vi "multicolor creation fast-3 only2ch(subvi).vi"(4 "on/off":bool[](array[boolean])=[TRUE, TRUE, FALSE, FALSE, FALSE, FALSE], 5 "colors":T1(array[cluster])=[{"color array"=[0, 16448250, 16448250, 16448250, 16776960, 16711680, 16448250, 16448250], "num of colors"=2, "max"=600.0, "min"=0.0}, {"color array"=[0, 16711680, 16776960, 16448250, 16776960, 16711680, 16448250, 16448250], "num of colors"=2, "max"=2000.0100000000002, "min"=100.0}, {"color array"=[0, 16711680, 16448250, 16448250, 16776960, 16711680, 16448250, 16448250], "num of colors"=2, "max"=12500.0, "min"=0.0}, {"color array"=[0, 255, 16448250, 16448250, 16776960, 16711680, 16448250, 16448250], "num of colors"=2, "max"=1.01, "min"=0.0}, {"color array"=[0, 65280, 16448250, 16448250, 16776960, 16711680, 16448250, 16448250], "num of colors"=3, "max"=1.0, "min"=0.0}, {"color array"=[0, 255, 16448250, 16448250, 16776960, 16711680, 16448250, 16448250], "num of colors"=2, "max"=1.0099999999999991, "min"=0.0}] {"min" step=0.01 format="%_2f"; "max" step=0.1 format="%_3f"}, 8 "fast/slow":bool=TRUE, 9 "img array in":dbl[][][](array[numeric])=array2x1024x1280[2621440 elements]) -> (1 "mixed img array":u32[][](array[numeric]))   [LabVIEW 2024]
panel:
  out "x-y 2":dbl
  out "Array":u32[][](array[numeric])
  out "x-y":dbl
  out "variant":variant
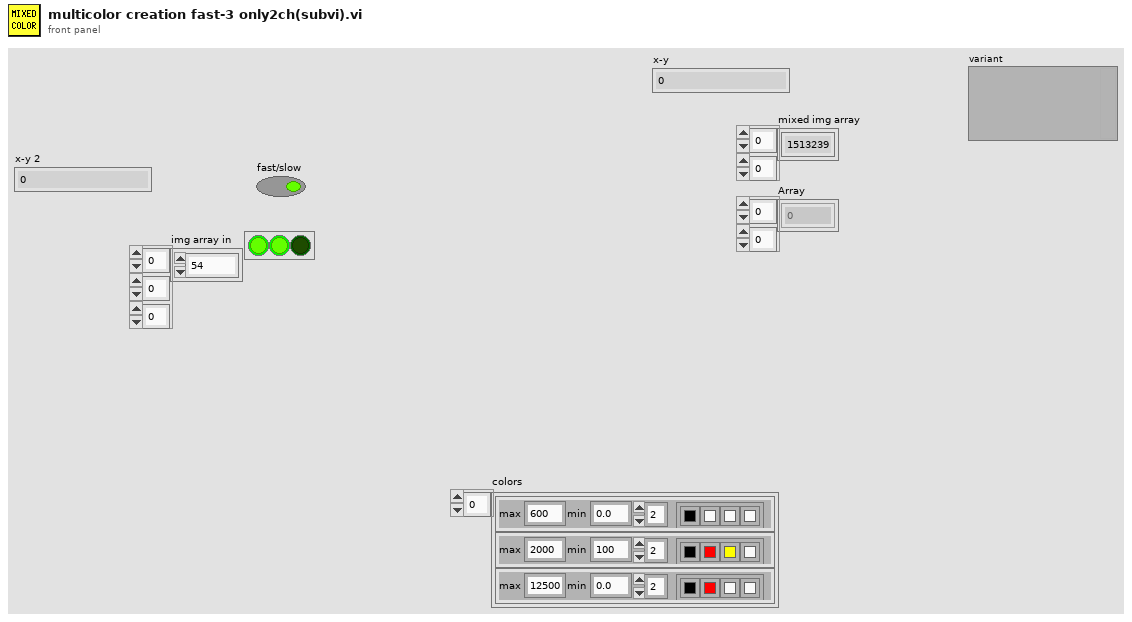
[diagram p1: front panel]
types:
  T1 = cluster{"color array":u32[], "num of colors":i32, "max":dbl, "min":dbl}[]
  T2 = cluster{"color array":u32[], "num of colors":i32, "max":dbl, "min":dbl}
  T3 = cluster{"color array":u32[], "num of colors":i32, "color array":u32[], "num of colors":i32}
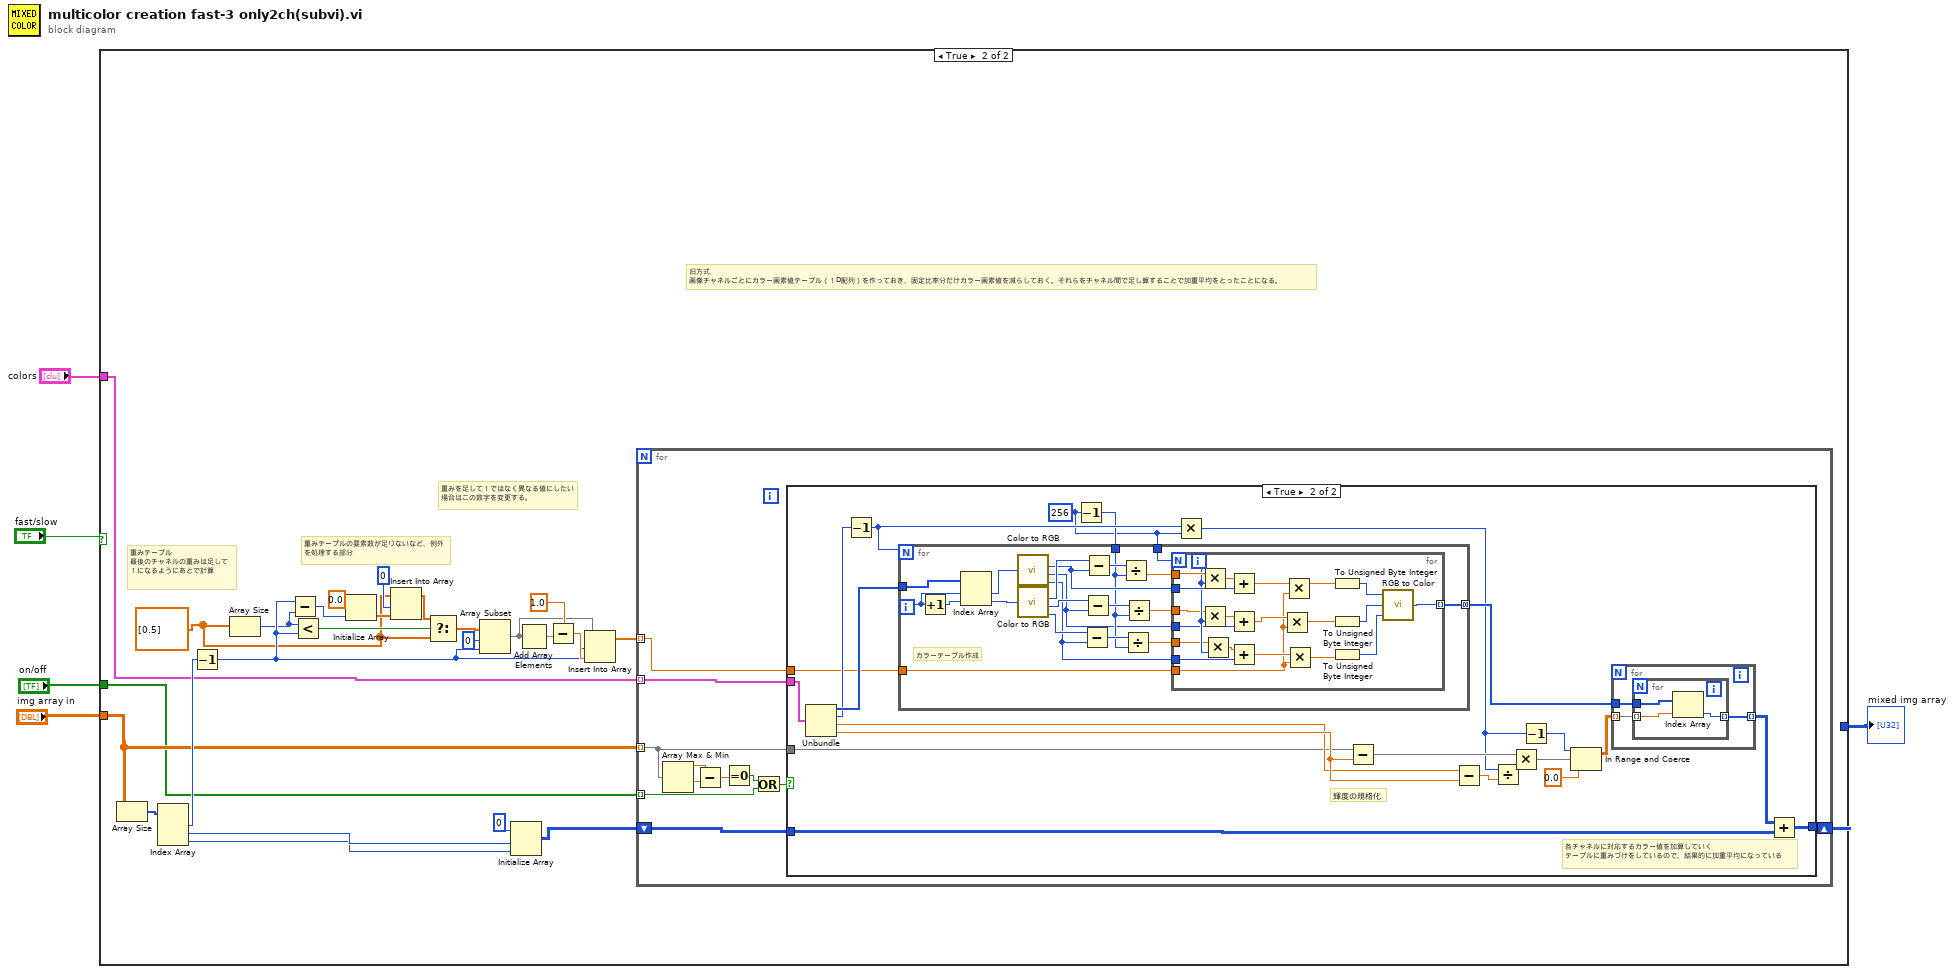
[diagram p0: block diagram]
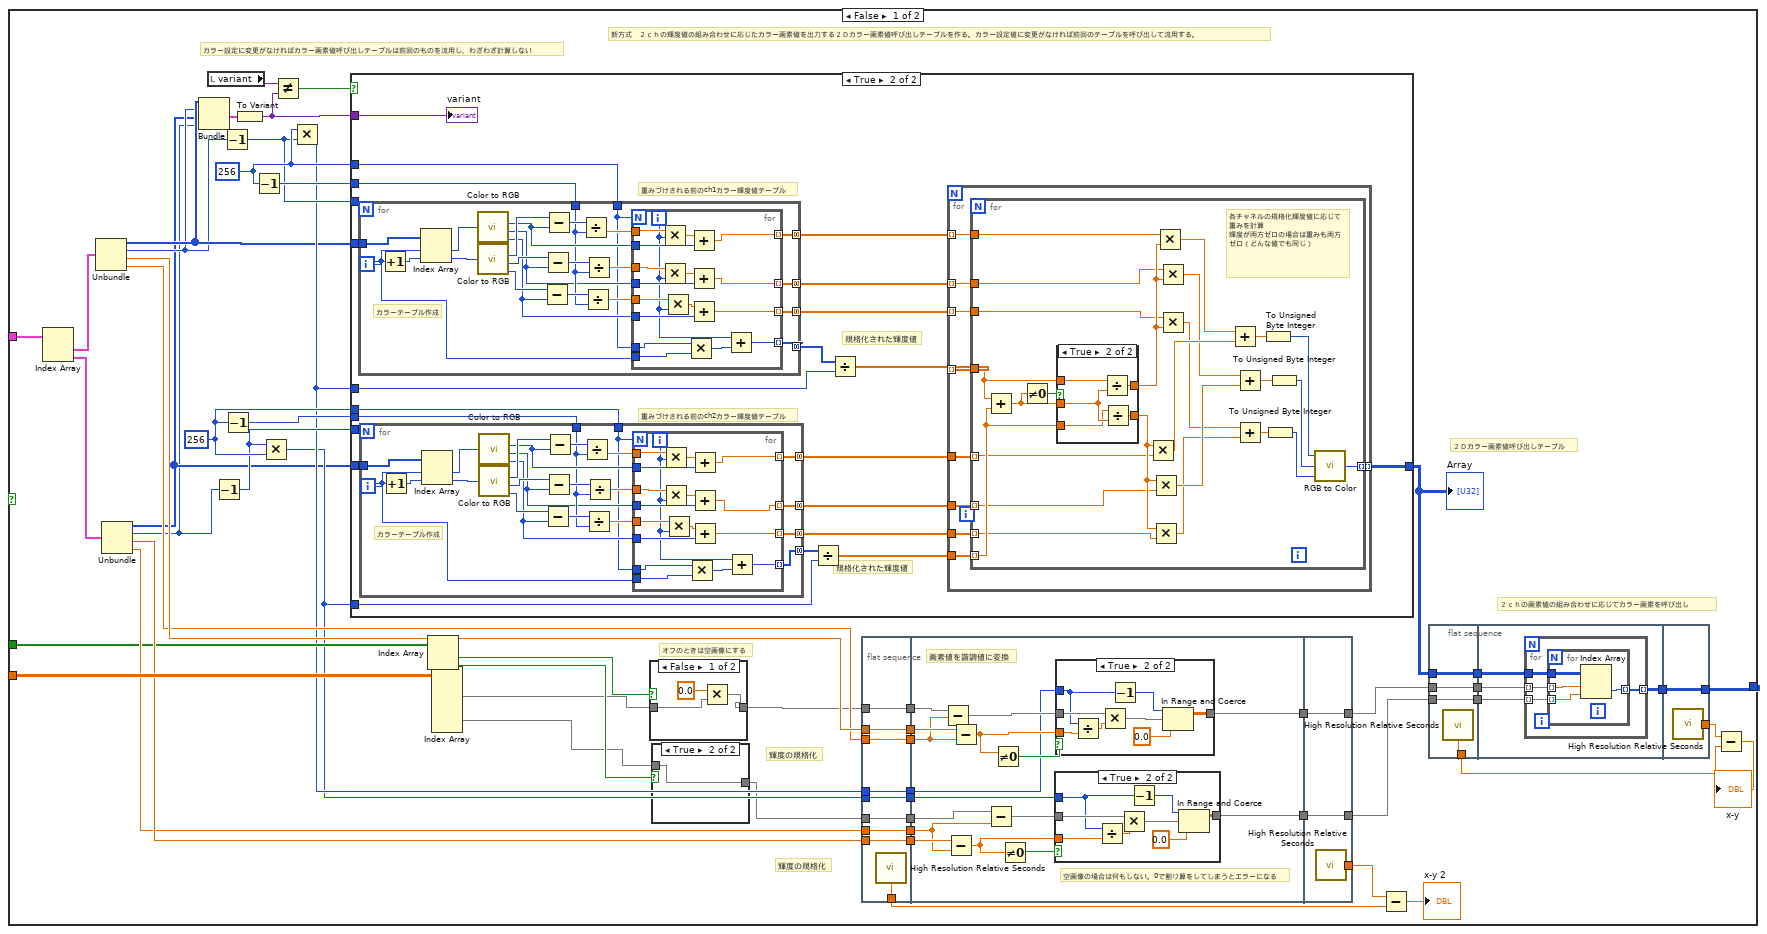
[diagram p2: hidden frame]
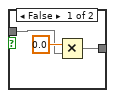
[diagram p3: hidden frame]
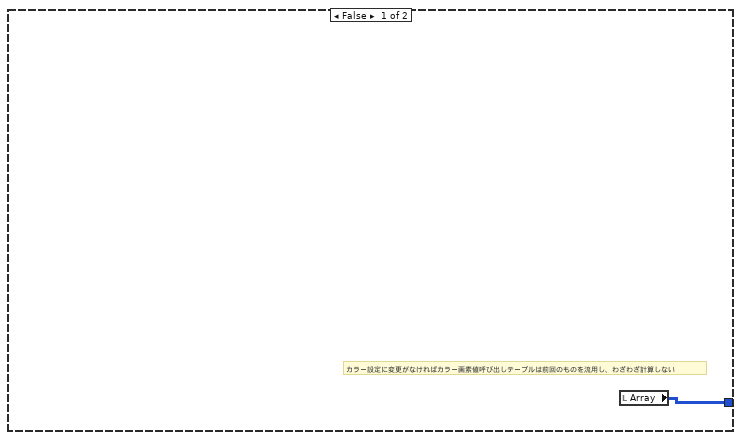
[diagram p7: hidden frame]
diagram:
  n1 = case shown="True" "fast/slow" {
    tunnel: "colors" -> [w46 w280]
    tunnel: "img array in" -> [w41 w279]
    tunnel: [w30 w281] -> w3
    tunnel: "on/off" -> [w29 w278]
    frame False {
      w36 = u16 256 ("y")
      w38 = u16 256 ("y")
      # "カラー設定に変更がなければカラー画素値呼び出しテーブルは前回のものを流用し、わざわざ計算しない"
      # "２ｃｈの画素値の組み合わせに応じてカラー画素を呼び出し"
      # "オフのときは空画像にする"
      # "２Ｄカラー画素値呼び出しテーブル"
      # "新方式　２ｃｈの輝度値の組み合わせに応じたカラー画素値を出力する２Ｄカラー画素値呼び出しテーブルを作る。カラー設定値に変更がなければ前回のテーブルを呼び出して流用する。"
      # "輝度の規格化"
      # "輝度の規格化"
      n2 = Index Array(array=w46) -> (element #1=w44:T2, element #2=w42:T2)  [unwired: 2 in]
      n3 = Unbundle(w44) -> ("color array"=w26:u32[], "num of colors"=w25:i32, "max"=w40:dbl, "min"=w39:dbl)
      n4 = Unbundle(w42) -> ("color array"=w24:u32[], "num of colors"=w23:i32, "max"=w34:dbl, "min"=w33:dbl)
      n5 = Bundle("color array"=w26, "num of colors"=w25, "color array"=w24, "num of colors"=w23) -> (w22:T3)  [unwired: 1 in]
      n6 = local read "variant"() -> (w20:variant)
      n7 = Decrement(x=w23) -> (x-1=w35:i32)
      n8 = Decrement(x=w25) -> (x-1=w37:i32)
      n9 = Decrement(x=w36) -> (x-1=w43:u16)
      n10 = To Variant(anything=w22) -> (Variant=w21:variant)
      n11 = Decrement(x=w38) -> (x-1=w45:u16)
      n12 = Multiply(x=w35, y=w36) -> (x*y=w27:i32)
      n13 = Not Equal?(x=w20, y=w21) -> (x != y?=w19:bool)
      n14 = Multiply(x=w38, y=w37) -> (x*y=w28:i32)
      n15 = case shown="True" w19 {
        tunnel: w26 -> [_ w155]
        tunnel: w45 -> [_ w154]
        tunnel: w43 -> [_ w151]
        tunnel: w24 -> [_ w150]
        tunnel: w38 -> [_ w141]
        tunnel: w37 -> [_ w140]
        tunnel: w36 -> [_ w139]
        tunnel: w35 -> [_ w138]
        tunnel: w28 -> [_ w137]
        tunnel: w27 -> [_ w136]
        tunnel: w21 -> [_ w135]
        tunnel: [w133 w134] -> w15
        frame False {
          # "カラー設定に変更がなければカラー画素値呼び出しテーブルは前回のものを流用し、わざわざ計算しない"
          n16 = local read "Array"() -> (w133:u32[][])
        }
        frame True {
          # "重みづけされる前のch2カラー輝度値テーブル"
          # "重みづけされる前のch1カラー輝度値テーブル"
          # "規格化された輝度値"
          # "規格化された輝度値"
          n17 = for {
            N: w140 -> [_]
            tunnel: w155 -> [w259]
            tunnel: w154 -> [w247]
            tunnel: w141 -> [w238]
            tunnel: [w242] -> w149 mode=concatenating
            tunnel: [w241] -> w148 mode=concatenating
            tunnel: [w240] -> w147 mode=concatenating
            tunnel: [w237] -> w153 mode=concatenating
            i -> [w239]
            # "カラーテーブル作成"
            n18 = Increment(x=w239) -> (x+1=w258:i32)
            n19 = Index Array(array=w259, index #1=w239, index #2=w258) -> (element #1=w257:u32, element #2=w256:u32)
            n20 = call <vilib>:"Color to RGB.vi"("Color"=w257) -> ("R"=w254:u8, "G"=w244:u8, "B"=w243:u8)  [unwired: 1 out]
            n21 = call <vilib>:"Color to RGB.vi"("Color"=w256) -> ("R"=w255:u8, "G"=w249:u8, "B"=w248:u8)  [unwired: 1 out]
            n22 = Subtract(x=w248, y=w243) -> (x-y=w250:u8)
            n23 = Subtract(x=w249, y=w244) -> (x-y=w251:u8)
            n24 = Subtract(x=w255, y=w254) -> (x-y=w253:u8)
            n25 = Divide(x=w253, y=w247) -> (x/y=w252:dbl)
            n26 = Divide(x=w250, y=w247) -> (x/y=w245:dbl)
            n27 = Divide(x=w251, y=w247) -> (x/y=w246:dbl)
            n28 = for {
              N: w238 -> [_]
              tunnel: w254 -> [w275]
              tunnel: w252 -> [w276]
              tunnel: w246 -> [w271]
              tunnel: w245 -> [w270]
              tunnel: w244 -> [w269]
              tunnel: w243 -> [w268]
              tunnel: [w262] -> w242 mode=indexing
              tunnel: [w261] -> w241 mode=indexing
              tunnel: [w260] -> w240 mode=indexing
              tunnel: w239 -> [w265]
              tunnel: w238 -> [w264]
              tunnel: [w263] -> w237 mode=indexing
              i -> [w267]
              n29 = Multiply(x=w276, y=w267) -> (x*y=w273:dbl)
              n30 = Multiply(x=w271, y=w267) -> (x*y=w274:dbl)
              n31 = Multiply(x=w270, y=w267) -> (x*y=w272:dbl)
              n32 = Multiply(x=w264, y=w265) -> (x*y=w266:i32)
              n33 = Add(x=w273, y=w275) -> (x+y=w262:dbl)
              n34 = Add(x=w274, y=w269) -> (x+y=w261:dbl)
              n35 = Add(x=w272, y=w268) -> (x+y=w260:dbl)
              n36 = Add(x=w267, y=w266) -> (x+y=w263:i32)
            }
          }
          n37 = for {
            N: w138 -> [_]
            tunnel: w150 -> [w219]
            tunnel: w151 -> [w207]
            tunnel: w139 -> [w198]
            tunnel: [w202] -> w146 mode=concatenating
            tunnel: [w201] -> w145 mode=concatenating
            tunnel: [w200] -> w144 mode=concatenating
            tunnel: [w197] -> w152 mode=concatenating
            i -> [w199]
            # "カラーテーブル作成"
            n38 = Increment(x=w199) -> (x+1=w218:i32)
            n39 = Index Array(array=w219, index #1=w199, index #2=w218) -> (element #1=w217:u32, element #2=w216:u32)
            n40 = call <vilib>:"Color to RGB.vi"("Color"=w217) -> ("R"=w214:u8, "G"=w204:u8, "B"=w203:u8)  [unwired: 1 out]
            n41 = call <vilib>:"Color to RGB.vi"("Color"=w216) -> ("R"=w215:u8, "G"=w209:u8, "B"=w208:u8)  [unwired: 1 out]
            n42 = Subtract(x=w208, y=w203) -> (x-y=w210:u8)
            n43 = Subtract(x=w209, y=w204) -> (x-y=w211:u8)
            n44 = Subtract(x=w215, y=w214) -> (x-y=w213:u8)
            n45 = Divide(x=w213, y=w207) -> (x/y=w212:dbl)
            n46 = Divide(x=w210, y=w207) -> (x/y=w205:dbl)
            n47 = Divide(x=w211, y=w207) -> (x/y=w206:dbl)
            n48 = for {
              N: w198 -> [_]
              tunnel: w214 -> [w235]
              tunnel: w212 -> [w236]
              tunnel: w206 -> [w231]
              tunnel: w205 -> [w230]
              tunnel: w204 -> [w229]
              tunnel: w203 -> [w228]
              tunnel: [w222] -> w202 mode=indexing
              tunnel: [w221] -> w201 mode=indexing
              tunnel: [w220] -> w200 mode=indexing
              tunnel: w199 -> [w225]
              tunnel: w198 -> [w224]
              tunnel: [w223] -> w197 mode=indexing
              i -> [w227]
              n49 = Multiply(x=w236, y=w227) -> (x*y=w233:dbl)
              n50 = Multiply(x=w231, y=w227) -> (x*y=w234:dbl)
              n51 = Multiply(x=w230, y=w227) -> (x*y=w232:dbl)
              n52 = Multiply(x=w224, y=w225) -> (x*y=w226:i32)
              n53 = Add(x=w233, y=w235) -> (x+y=w222:dbl)
              n54 = Add(x=w234, y=w229) -> (x+y=w221:dbl)
              n55 = Add(x=w232, y=w228) -> (x+y=w220:dbl)
              n56 = Add(x=w227, y=w226) -> (x+y=w223:i32)
            }
          }
          n57 = Divide(x=w152, y=w136) -> (x/y=w143:dbl[])
          n58 = Divide(x=w153, y=w137) -> (x/y=w142:dbl[])
          n59 = for {
            tunnel: w149 -> [w157] mode=indexing
            tunnel: w148 -> [w158] mode=indexing
            tunnel: w147 -> [w159] mode=indexing
            tunnel: w146 -> [w164]
            tunnel: w145 -> [w163]
            tunnel: w144 -> [w162]
            tunnel: w143 -> [w161]
            tunnel: w142 -> [w160] mode=indexing
            tunnel: [w156] -> w134 mode=indexing
            n60 = for {
              tunnel: w164 -> [w186] mode=indexing
              tunnel: w163 -> [w185] mode=indexing
              tunnel: w162 -> [w184] mode=indexing
              tunnel: w161 -> [w188] mode=indexing
              tunnel: w160 -> [w189]
              tunnel: w159 -> [w180]
              tunnel: w158 -> [w181]
              tunnel: w157 -> [w182]
              tunnel: [w165] -> w156 mode=indexing
              # "各チャネルの規格化輝度値に応じて重みを計算\n輝度が両方ゼロの場合は重みも両方ゼロ（どんな値でも同じ）"
              n61 = Add(x=w189, y=w188) -> (x+y=w169:dbl)
              n62 = Not Equal To 0?(x=w169) -> (x != 0?=w170:bool)
              n63 = case shown="True" w170 {
                tunnel: w169 -> [_ w196]
                tunnel: w189 -> [w191 w195]
                tunnel: w188 -> [w190 w194]
                tunnel: [w190 w193] -> w187
                tunnel: [w191 w192] -> w183
                frame False {
                }
                frame True {
                  n64 = Divide(x=w195, y=w196) -> (x/y=w192:dbl)
                  n65 = Divide(x=w194, y=w196) -> (x/y=w193:dbl)
                }
              }
              n66 = Multiply(x=w187, y=w186) -> (x*y=w178:dbl)
              n67 = Multiply(x=w187, y=w185) -> (x*y=w176:dbl)
              n68 = Multiply(x=w187, y=w184) -> (x*y=w174:dbl)
              n69 = Multiply(x=w182, y=w183) -> (x*y=w179:dbl)
              n70 = Multiply(x=w181, y=w183) -> (x*y=w177:dbl)
              n71 = Multiply(x=w180, y=w183) -> (x*y=w175:dbl)
              n72 = Add(x=w179, y=w178) -> (x+y=w173:dbl)
              n73 = Add(x=w177, y=w176) -> (x+y=w172:dbl)
              n74 = Add(x=w175, y=w174) -> (x+y=w171:dbl)
              n75 = To Unsigned Byte Integer(number=w173) -> (unsigned 8bit integer=w168:u8)
              n76 = To Unsigned Byte Integer(number=w171) -> (unsigned 8bit integer=w166:u8)
              n77 = To Unsigned Byte Integer(number=w172) -> (unsigned 8bit integer=w167:u8)
              n78 = call <vilib>:"RGB to Color.vi"("B"=w166, "G"=w167, "R"=w168) -> ("Color"=w165:u32)
            }
          }
          "variant" <- w135
        }
      }
      "Array" <- w15
      n79 = Index Array(array=w29) -> (element #1=w11:bool, element #2=w10:bool)  [unwired: 2 in]
      n80 = Index Array(array=w41) -> (element #1=w9:dbl[][], element #2=w7:dbl[][])  [unwired: 6 in]
      n81 = case shown="False" w11 {
        tunnel: w9 -> [w66 w68]
        tunnel: [w65 w68] -> w8
        frame False {
          n82 = Multiply(x=0.0, y=w66) -> (x*y=w65:dbl[][])
        }
        frame True {
        }
      }
      n83 = case shown="True" w10 {
        tunnel: w7 -> [w62 w64]
        tunnel: [w61 w64] -> w6
        frame False {
          n84 = Multiply(x=0.0, y=w62) -> (x*y=w61:dbl[][])
        }
        frame True {
        }
      }
      n85 = flat-sequence {
        tunnel: w27 -> [w70]
        tunnel: w28 -> [w71]
        tunnel: w6 -> [w72]
        tunnel: w8 -> [w73]
        tunnel: w33 -> [w74]
        tunnel: w34 -> [w75]
        tunnel: w39 -> [w76]
        tunnel: w40 -> [w77]
        tunnel: [w77] -> w56
        tunnel: [w76] -> w55
        tunnel: [w75] -> w54
        tunnel: [w74] -> w53
        tunnel: [w73] -> w52
        tunnel: [w72] -> w51
        tunnel: [w71] -> w50
        tunnel: [w70] -> w49
        tunnel: [w69] -> w12
        tunnel: [w87] -> w48
        tunnel: [w86] -> w47
        tunnel: w56 -> [w92]
        tunnel: w55 -> [w91]
        tunnel: w54 -> [w89]
        tunnel: w53 -> [w88]
        tunnel: w52 -> [w81]
        tunnel: w51 -> [w80]
        tunnel: w50 -> [w79]
        tunnel: w49 -> [w78]
        tunnel: [w113] -> w31
        tunnel: [w114] -> w32
        tunnel: w48 -> [w114]
        tunnel: w47 -> [w113]
        tunnel: [w112] -> w13
        frame #0 {
          n86 = call <vilib>:"High Resolution Relative Seconds.vi"() -> ("relative seconds"=w69:dbl)
        }
        frame #1 {
          # "空画像の場合は何もしない。0で割り算をしてしまうとエラーになる"
          # "画素値を諧調値に変換"
          n87 = Subtract(x=w81, y=w91) -> (x-y=w93:dbl[][])
          n88 = Subtract(x=w89, y=w88) -> (x-y=w83:dbl)
          n89 = Subtract(x=w92, y=w91) -> (x-y=w85:dbl)
          n90 = Subtract(x=w80, y=w88) -> (x-y=w90:dbl[][])
          n91 = Not Equal To 0?(x=w85) -> (x != 0?=w84:bool)
          n92 = Not Equal To 0?(x=w83) -> (x != 0?=w82:bool)
          n93 = case shown="True" w82 {
            tunnel: w83 -> [_ w101]
            tunnel: w90 -> [w94 w99]
            tunnel: w78 -> [_ w96]
            tunnel: [w94 w95] -> w86
            frame False {
            }
            frame True {
              n94 = Divide(x=w96, y=w101) -> (x/y=w100:dbl)
              n95 = Multiply(x=w99, y=w100) -> (x*y=w102:dbl[][])
              n96 = Decrement(x=w96) -> (x-1=w97:i32)
              n97 = In Range and Coerce(upper limit=w97, x=w102, lower limit=0.0) -> (coerced(x)=w95:dbl[][])  [unwired: 1 out]
            }
          }
          n98 = case shown="True" w84 {
            tunnel: w93 -> [w103 w109]
            tunnel: w85 -> [_ w107]
            tunnel: w79 -> [_ w105]
            tunnel: [w103 w104] -> w87
            frame False {
            }
            frame True {
              n99 = Divide(x=w105, y=w107) -> (x/y=w108:dbl)
              n100 = Multiply(x=w109, y=w108) -> (x*y=w106:dbl[][])
              n101 = Decrement(x=w105) -> (x-1=w111:i32)
              n102 = In Range and Coerce(upper limit=w111, x=w106, lower limit=0.0) -> (coerced(x)=w104:dbl[][])  [unwired: 1 out]
            }
          }
        }
        frame #2 {
          n103 = call <vilib>:"High Resolution Relative Seconds.vi"() -> ("relative seconds"=w112:dbl)
        }
      }
      n104 = Subtract(x=w13, y=w12) -> (x-y=→"x-y 2":dbl)
      n105 = flat-sequence {
        tunnel: w15 -> [w116]
        tunnel: w31 -> [w117]
        tunnel: w32 -> [w118]
        tunnel: [w118] -> w60
        tunnel: [w117] -> w59
        tunnel: [w116] -> w58
        tunnel: [w115] -> w17
        tunnel: [w119] -> w57
        tunnel: w60 -> [w122]
        tunnel: w59 -> [w121]
        tunnel: w58 -> [w120]
        tunnel: [w132] -> w30
        tunnel: w57 -> [w132]
        tunnel: [w131] -> w18
        frame #0 {
          n106 = call <vilib>:"High Resolution Relative Seconds.vi"() -> ("relative seconds"=w115:dbl)
        }
        frame #1 {
          n107 = for {
            tunnel: w122 -> [w126] mode=indexing
            tunnel: w121 -> [w125] mode=indexing
            tunnel: w120 -> [w124]
            tunnel: [w123] -> w119 mode=indexing
            n108 = for {
              tunnel: w126 -> [w129] mode=indexing
              tunnel: w125 -> [w128] mode=indexing
              tunnel: w124 -> [w130]
              tunnel: [w127] -> w123 mode=indexing
              n109 = Index Array(array=w130, index (row)=w129, index (col)=w128) -> (element=w127:u32)
            }
          }
        }
        frame #2 {
          n110 = call <vilib>:"High Resolution Relative Seconds.vi"() -> ("relative seconds"=w131:dbl)
        }
      }
      n111 = Subtract(x=w18, y=w17) -> (x-y=→"x-y":dbl)
    }
    frame True {
      w277 = dbl[] [0.5] ("array")
      # "重みを足して１ではなく異なる値にしたい場合はこの数字を変更する。"
      # "重みテーブル\n最後のチャネルの重みは足して１になるようにあとで計算"
      # "重みテーブルの要素数が足りないなど、例外を処理する部分"
      # "旧方式\n画像チャネルごとにカラー画素値テーブル（１D配列）を作っておき、固定比率分だけカラー画素値を減らしておく。それらをチャネル間で足し算することで加重平均をとったことになる。"
      n112 = Array Size(array=w279) -> (size(s)=w302:i32[])
      n113 = Index Array(array=w302) -> (element #1=w297:i32, element #2=w299:i32, element #3=w298:i32)  [unwired: 3 in]
      n114 = Decrement(x=w297) -> (x-1=w290:i32)
      n115 = Array Size(array=w277) -> (size(s)=w289:i32)
      n116 = Subtract(x=w290, y=w289) -> (x-y=w288:i32)
      n117 = Less?(x=w289, y=w290) -> (x < y?=w291:bool)
      n118 = Initialize Array(0.0 ("element"), w288) -> (w286:dbl[])
      n119 = Insert Into Array(array=w277, index=0, new element=w286) -> (w284:dbl[])
      n120 = Select(t=w284, s=w291, f=w277) -> (s? t:f=w283:dbl[])
      n121 = Array Subset(array=w283, index=0, length=w290) -> (w282:dbl[])
      n122 = Initialize Array(u32 0, w299, w298) -> (w300:u32[][])
      n123 = Add Array Elements(numeric array=w282) -> (sum=w295:dbl)
      n124 = Subtract(x=1.0, y=w295) -> (x-y=w293:dbl)
      n125 = Insert Into Array(array=w282, index=w290, new element=w293) -> (w292:dbl[])
      n126 = for {
        tunnel: w280 -> [w313] mode=indexing
        tunnel: w279 -> [w312] mode=indexing
        tunnel: w278 -> [w311] mode=indexing
        shift-right: [w310] -> w281
        shift-left: w300 -> [w309]
        tunnel: w292 -> [w303] mode=indexing
        n127 = Array Max & Min(array=w312) -> (max value=w308:dbl, min value=w307:dbl)  [unwired: 2 out]
        n128 = Subtract(x=w308, y=w307) -> (x-y=w306:dbl)
        n129 = Equal To 0?(x=w306) -> (x = 0?=w305:bool)
        n130 = Or(x=w305, y=w311) -> (x .or. y?=w304:bool)
        n131 = case shown="True" w304 {
          tunnel: w313 -> [_ w334]
          tunnel: w312 -> [_ w333]
          tunnel: [w314 w332] -> w310
          tunnel: w309 -> [w314 w331]
          tunnel: w303 -> [_ w319]
          frame False {
          }
          frame True {
            w323 = u16 256 ("y")
            # "輝度の規格化"
            # "各チャネルに対応するカラー値を加算していく\nテーブルに重みづけをしているので、結果的に加重平均になっている"
            n132 = Unbundle(w334) -> ("color array"=w330:u32[], "num of colors"=w329:i32, "max"=w335:dbl, "min"=w336:dbl)
            n133 = Decrement(x=w329) -> (x-1=w325:i32)
            n134 = Decrement(x=w323) -> (x-1=w324:u16)
            n135 = for {
              N: w325 -> [_]
              tunnel: w330 -> [w363]
              tunnel: w324 -> [w350]
              tunnel: w323 -> [w349]
              tunnel: [w346] -> w328 mode=concatenating
              tunnel: w319 -> [w343]
              i -> [w361]
              # "カラーテーブル作成"
              n136 = Increment(x=w361) -> (x+1=w362:i32)
              n137 = Index Array(array=w363, index #1=w361, index #2=w362) -> (element #1=w360:u32, element #2=w359:u32)
              n138 = call <vilib>:"Color to RGB.vi"("Color"=w360) -> ("R"=w357:u8, "G"=w345:u8, "B"=w344:u8)  [unwired: 1 out]
              n139 = call <vilib>:"Color to RGB.vi"("Color"=w359) -> ("R"=w358:u8, "G"=w352:u8, "B"=w351:u8)  [unwired: 1 out]
              n140 = Subtract(x=w351, y=w344) -> (x-y=w353:u8)
              n141 = Subtract(x=w352, y=w345) -> (x-y=w354:u8)
              n142 = Subtract(x=w358, y=w357) -> (x-y=w356:u8)
              n143 = Divide(x=w356, y=w350) -> (x/y=w355:dbl)
              n144 = Divide(x=w353, y=w350) -> (x/y=w347:dbl)
              n145 = Divide(x=w354, y=w350) -> (x/y=w348:dbl)
              n146 = for {
                N: w349 -> [_]
                tunnel: w357 -> [w383]
                tunnel: w355 -> [w384]
                tunnel: w348 -> [w377]
                tunnel: w347 -> [w376]
                tunnel: [w375] -> w346 mode=indexing
                tunnel: w345 -> [w374]
                tunnel: w344 -> [w373]
                tunnel: w343 -> [w364]
                i -> [w378]
                n147 = Multiply(x=w384, y=w378) -> (x*y=w380:dbl)
                n148 = Multiply(x=w377, y=w378) -> (x*y=w381:dbl)
                n149 = Multiply(x=w376, y=w378) -> (x*y=w379:dbl)
                n150 = Add(x=w380, y=w383) -> (x+y=w382:dbl)
                n151 = Add(x=w381, y=w374) -> (x+y=w366:dbl)
                n152 = Add(x=w379, y=w373) -> (x+y=w365:dbl)
                n153 = Multiply(x=w366, y=w364) -> (x*y=w368:dbl)
                n154 = Multiply(x=w382, y=w364) -> (x*y=w369:dbl)
                n155 = Multiply(x=w365, y=w364) -> (x*y=w367:dbl)
                n156 = To Unsigned Byte Integer(number=w369) -> (unsigned 8bit integer=w372:u8)
                n157 = To Unsigned Byte Integer(number=w368) -> (unsigned 8bit integer=w371:u8)
                n158 = To Unsigned Byte Integer(number=w367) -> (unsigned 8bit integer=w370:u8)
                n159 = call <vilib>:"RGB to Color.vi"("B"=w370, "G"=w371, "R"=w372) -> ("Color"=w375:u32)
              }
            }
            n160 = Multiply(x=w325, y=w323) -> (x*y=w316:i32)
            n161 = Subtract(x=w333, y=w336) -> (x-y=w320:dbl[][])
            n162 = Subtract(x=w335, y=w336) -> (x-y=w322:dbl)
            n163 = Divide(x=w316, y=w322) -> (x/y=w321:dbl)
            n164 = Multiply(x=w320, y=w321) -> (x*y=w327:dbl[][])
            n165 = Decrement(x=w316) -> (x-1=w315:i32)
            n166 = In Range and Coerce(upper limit=w315, x=w327, lower limit=0.0) -> (coerced(x)=w318:dbl[][])  [unwired: 1 out]
            n167 = for {
              tunnel: w328 -> [w339]
              tunnel: w318 -> [w338] mode=indexing
              tunnel: [w337] -> w326 mode=indexing
              n168 = for {
                tunnel: w339 -> [w342]
                tunnel: w338 -> [w340] mode=indexing
                tunnel: [w341] -> w337 mode=indexing
                n169 = Index Array(array=w342, index=w340) -> (element=w341:u32)
              }
            }
            n170 = Add(x=w326, y=w331) -> (x+y=w332:u32[][])
          }
        }
      }
    }
  }
  "mixed img array" <- w3
